vi "Dashboard Main.vi"() -> ()   [LabVIEW 2019]
uses:
  <vilib>/Rock Robotics/Network Tables/NT Read Numeric Array.vi
  <vilib>/Rock Robotics/Network Tables/NT Read String.vi
  <vilib>/Rock Robotics/Network Tables/NT Read Number.vi
  <vilib>/Rock Robotics/Network Tables/NT Read Boolean.vi
  <vilib>/Rock Robotics/Network Tables/NT Write Number.vi
panel:
  out "Camera Perf":string
  in  "Camera Settings":T1={"Frame Rate"=30, "Compression"=30, "Size"=1, "DB Camera Config"=FALSE} {"Frame Rate" scale=1.0..30.0; "Compression" scale=100.0..-1.0; "Size" items=["640x480", "320x240", "160x120"]}
  in  "TCP":refnum<k5>
  out "Robot IP":string
  in  "Dashboard Tab":T2(tab)
  in  "Select Auto":string(combo)="Select Autonomous ..."
  out "NT Connection":bool
  out "MotorChart R":cluster{"Numeric":dbl, "Numeric":dbl}(graph)
  out "MotorChart L":cluster{"Numeric":dbl, "Numeric":dbl}(graph)
  out "MotorSliders R":cluster{"MotorSlide1":dbl, "MotorSlide2":dbl} {"MotorSlide2" scale=-1.0..1.0 scale format="%#_2e"; "MotorSlide1" scale=-1.0..1.0 scale format="%#_2e"}
  out "MotorSliders L":cluster{"MotorSlide1":dbl, "MotorSlide2":dbl} {"MotorSlide2" scale=-1.0..1.0 scale format="%#_2e"; "MotorSlide1" scale=-1.0..1.0 scale format="%#_2e"}
  out "JS1 Z":dbl(slide) scale=-1.0..1.0 scale format="%#_2e"
  out "JS1 Graph":cluster{"X":dbl, "Y":dbl}[](graph)
  out "JS1 Buttons":T3
  out "JS2 Z":dbl(slide) scale=-1.0..1.0 scale format="%#_2e"
  out "JS2 Graph":cluster{"X":dbl, "Y":dbl}[](graph)
  out "JS2 Buttons":T3
  out "Mode":T4(ring)=enum."Auto Disabled"
  in  "Camera Name 2":string(combo)="No Camera Selection"
  out "Camera Image 2":T5(plugin-control)
  out "Target Spotted":bool
  out "Color Box":u32(colorbox)
  out "New Center Y":dbl
  out "New Center X":dbl
  out "y change":dbl
  out "Top Left Y":dbl
  out "Bottom Right Y":dbl
  out "Bottom Right X":dbl
  out "Top left X":dbl
  out "x change":dbl
  out "full angle":dbl
  in  "RectHeight":dbl
  in  "RectWidth":dbl
  in  "RectAngle":dbl
  in  "RectY":dbl
  in  "RectX":dbl
  out "Distance Formula 2":dbl
  out "Distance Formula 1":dbl
  out "Bottom Left Y":dbl
  out "Bottom Left X":dbl
  out "Top Right X":dbl
  out "Top Right Y":dbl
  out "New Full Angle":dbl
  out "2nd Y Change":dbl
  out "2nd X Change":dbl
  out "Final Center Y":dbl
  out "Final Center X":dbl
  out "Robot Angle":dbl
  out "Right Target":dbl
  out "Left Target":dbl
  out "Average Distance":dbl
  out "Right Distance":dbl
  out "Left Distance":dbl
  out "Right Speed":dbl
  out "Average Speed":dbl
  out "Left Speed":dbl
  out "Left":dbl[](graph)
  out "Right":dbl[](graph)
  out "Current Filter":T6 {"Value" scale=0.0..255.0; "Saturation" scale=0.0..255.0; "Hue" scale=0.0..255.0}
  in  "Update Filter":bool
  in  "New Filter":T6 {"Value" scale=0.0..255.0; "Saturation" scale=0.0..255.0; "Hue" scale=0.0..255.0}
  out "RectX":dbl
  out "RectY":dbl
  out "RectAngle":dbl
  out "RectWidth":dbl
  out "RectHeight":dbl
  out "left y":dbl
  out "right y":dbl
  out "right x":dbl
  out "left x":dbl
  out "right dmd":dbl format="%10.0f"
  out "lft dmd":dbl format="%10.0f"
  in  "Demand":bool
  in  "C Height":dbl format="%10.0f"
  in  "Update":bool
  in  "Kd":dbl format="%10.0f"
  in  "Ki":dbl format="%10.0f"
  in  "Kp":dbl format="%10.0f"
  in  "Kf":dbl format="%10.0f"
  out "Right Speed 2":dbl format="%10.0f"
  out "Left Speed 2":dbl format="%10.0f"
  out "Waveform Chart":dbl[](graph)
  in  "Right Dmd":dbl format="%10.0f"
  in  "Left Dmd":dbl format="%10.0f"
  out "Tree":string(tree)
  out "Camera Image":T5(plugin-control)
  out "Background":bool
  in  "Camera Name":string(combo)="No Camera Selection"
  # "HW"
  # "Joysticks"
  # "Drive Motors"
  # "Front"
  # "Right"
  # "Left"
  # "Back"
  # "Target Spotted"
  # "Color Sensor 90 Degree Color"
  # "Left"
  # "Right"
  # "Average"
  # "Speed"
  # "Target Speed"
  # "Distance"
  # "Robot Angle"
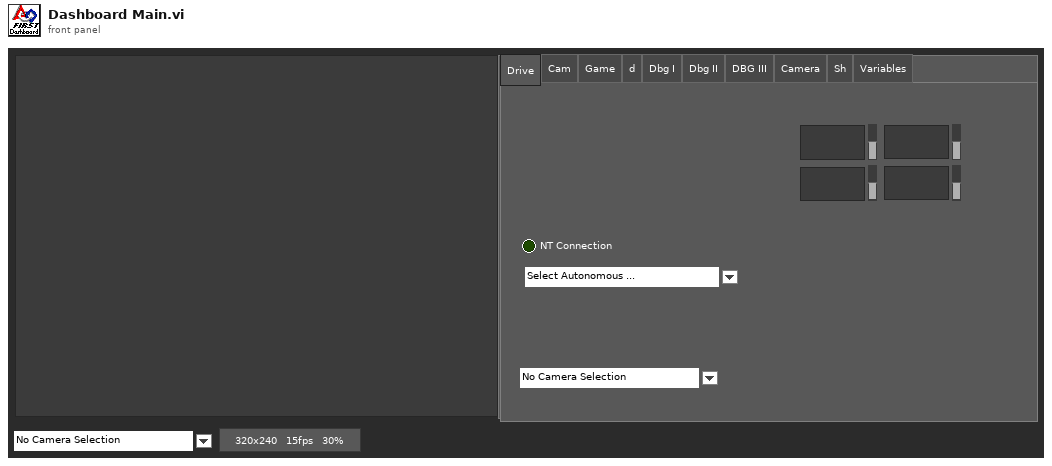
[diagram p1: front panel]
types:
  T1 = cluster{"Frame Rate":i32, "Compression":i32, "Size":u16, "DB Camera Config":bool}
  T2 = enum32{"Drive", "Cam", "Game", "d", "Dbg I", "Dbg II", "DBG III", "Camera", "Sh", "Variables"}
  T3 = cluster{bool, bool, bool, bool, bool, bool, bool, bool, bool, bool, bool, bool}
  T4 = enum8{"Tele-Op Disabled", "Tele-Op Enabled", "Auto Disabled", "Auto Enabled", "Test Disabled", "Test Enabled", "Disconnected", "No Code", "E-Stop"}
  T5 = typedef "IMAQ Image.ctl" = refnum<image>
  T6 = cluster{"Hue":cluster{dbl, dbl}, "Saturation":cluster{dbl, dbl}, "Value":cluster{dbl, dbl}}
  T7 = typedef "Image Type" = u32
  T8 = cluster{"Save Path":path, "Interval (s)":dbl, "Keep":i32}
  T9 = cluster{"Camera Image":refnum<vi>, "Dashboard Tab":refnum<vi>, "Background":refnum<vi>, "Tree":refnum<vi>, "Camera Settings":refnum<vi>, "Camera Name":refnum<vi>, "Camera Perf":refnum<vi>}
  T10 = cluster{"Shift":bool, "Ctrl":bool, "Alt":bool, "Cmd":bool, "Opt":bool}
  T11 = cluster{"Camera Name":string, "Camera File Name":string, "Saved DB Images Info":cluster{"Save Path":path, "Interval (s)":dbl, "Keep":i32}}
  T12 = cluster{"left x":dbl, "left y":dbl, "right x":dbl, "right y":dbl}
  T13 = cluster{cluster{dbl, dbl}, cluster{dbl, dbl}, cluster{dbl, dbl}}
  T14 = cluster{"left x":dbl, "right y":dbl, "right x":dbl, "left y":dbl}
  T15 = cluster{"Camera Name 2":string, string, "Saved DB Images Info":cluster{"Save Path":path, "Interval (s)":dbl, "Keep":i32}}
  T16 = cluster{"Error Strings":string, "Disable Counts":cluster{u16, u16}, "Rail Faults":cluster{u16, u16, u16}, "Robot IP":string, "DB Mode":u8, "Event Info":cluster{"Name":string, "Type":u8, "Number":u16, "Replay":u8}}
  T17 = cluster{"Storage":cluster{"Disk Free":u64, "RAM Block":u32, "RAM free":u32}, "CPU Utilization":cluster{"CPU % ISR":sgl, "CPU % Time Crit":sgl, "CPU % Timed Str":sgl, "CPU % High":sgl, "CPU % Above":sgl, "CPU % Normal":sgl, "CPU % Low":sgl}, "CAN":cluster{"% Bus Utilization":sgl, "Bus Off Cnt":u32, "TX_FIFO Full Cnt":u32, "Receive Error Cnt":u8, "Transmit Error Cnt":u8}, "HID":cluster{"HID Outputs":u32, "Rumble Low":u16, "Rumble High":u16}[]}
  T18 = cluster{"Status bits":cluster{"Test Mode":bool, "Autonomous":bool, "Enabled":bool, "Code Start":bool, "Brownout":bool, "Reserved 2":bool, "Reserved 3":bool, "E-Stop":bool}, "Code Trace":cluster{"Disabled":bool, "TeleOp":bool, "Auto":bool, "Test":bool}, "Controller Type":enum16{"unknown", "cRIO", "roboRio"}, "Code?":enum16{"unknown", "noCode", "code"}, "Battery V":dbl}
  T19 = cluster{"Control Bits":cluster{"TestMode":bool, "Autonomous":bool, "Enabled":bool, "FMS Present":bool, bool, bool, bool, "E-Stop":bool}, "Team Station ":u8, "Countdown":sgl, "Joystick Values":cluster{"Axes":dbl[], "Buttons":bool[], "POVs":i16[]}[]}
  T20 = cluster{"Axes":dbl[], "Buttons":bool[], "POVs":i16[]}[]
  T21 = cluster{"Axes":dbl[], "Buttons":bool[], "POVs":i16[]}
  T22 = cluster{"Buttons[0]":bool, "Buttons[1]":bool, "Buttons[2]":bool, "Buttons[3]":bool, "Buttons[4]":bool, "Buttons[5]":bool, "Buttons[6]":bool, "Buttons[7]":bool, "Buttons[8]":bool, "Buttons[9]":bool, "Buttons[10]":bool, "Buttons[11]":bool}
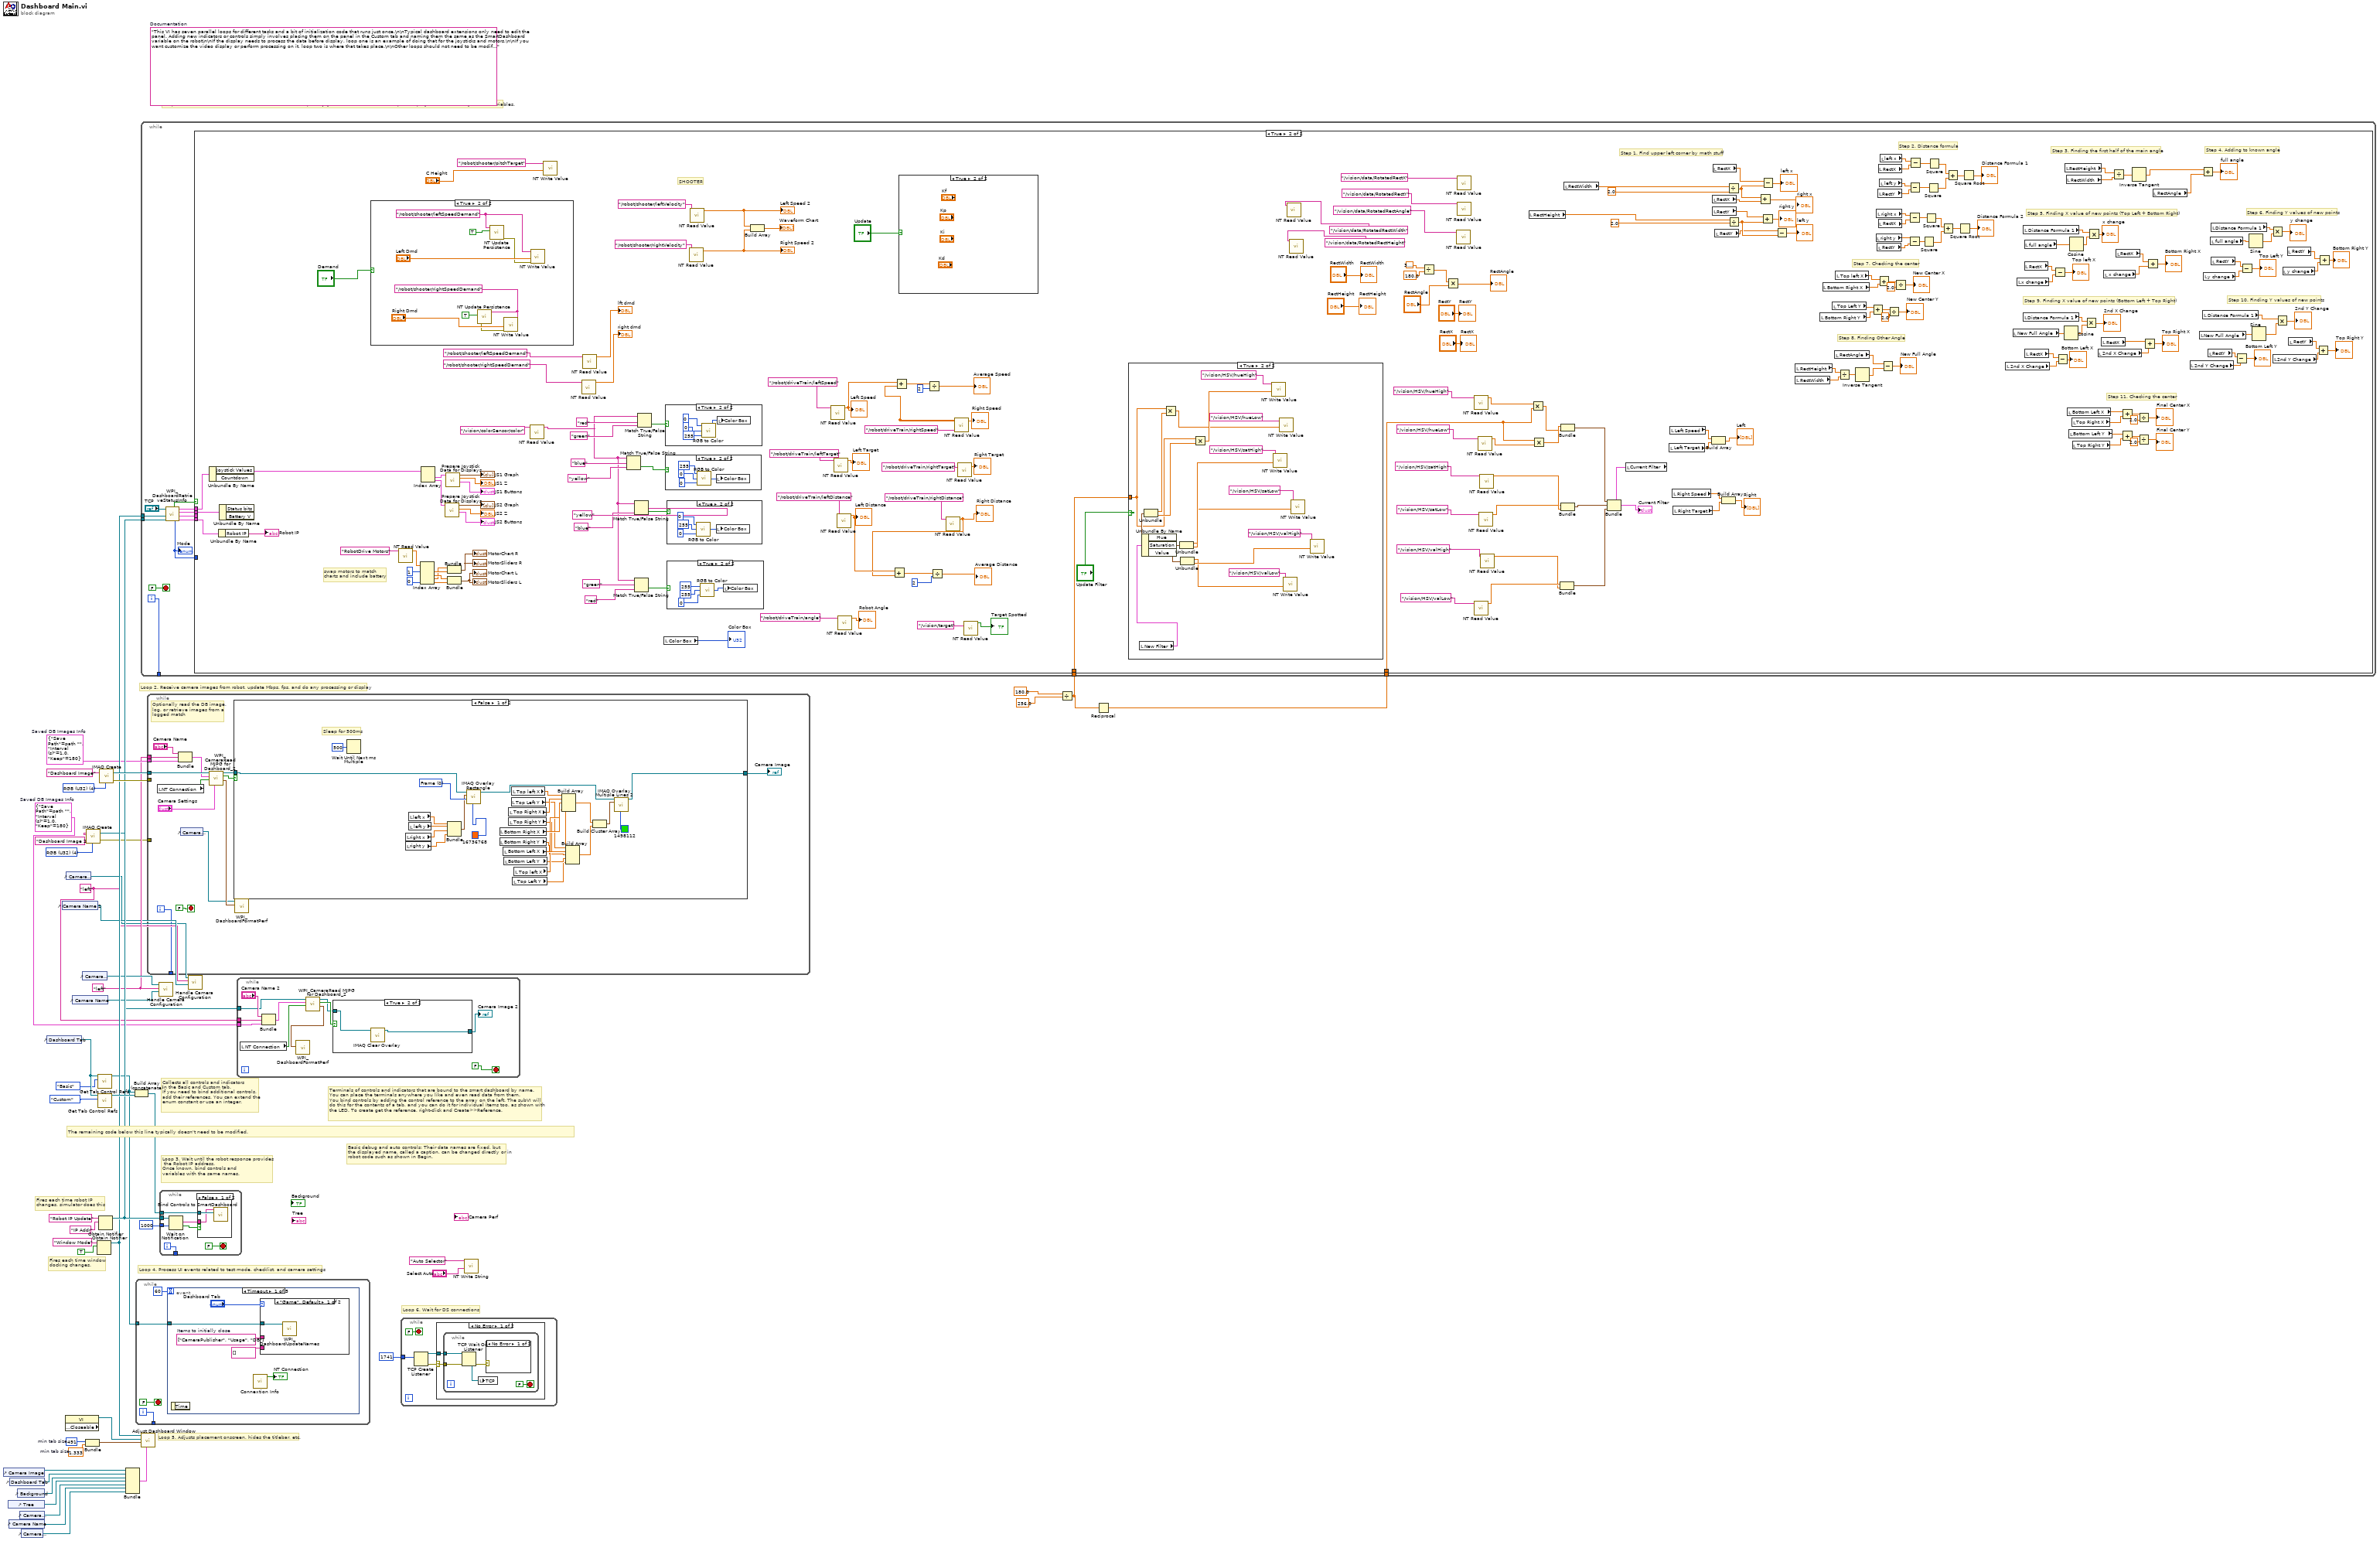
[diagram p0: block diagram]
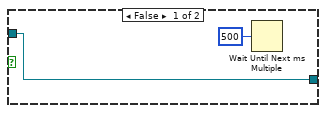
[diagram p2: hidden frame]
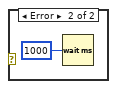
[diagram p3: hidden frame]
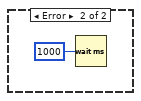
[diagram p4: hidden frame]
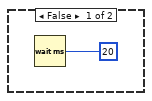
[diagram p5: hidden frame]
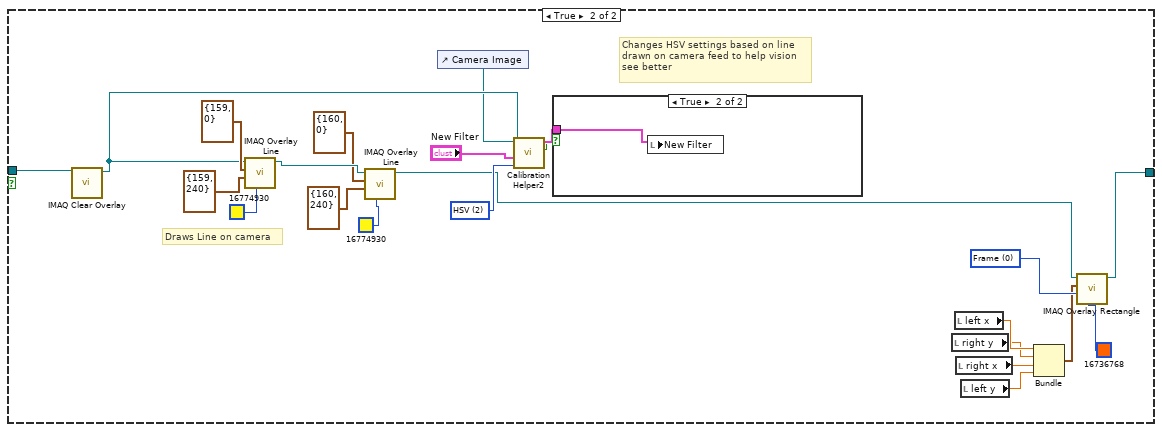
[diagram p14: hidden frame]
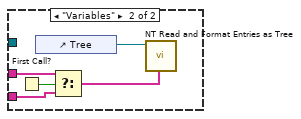
[diagram p16: hidden frame]
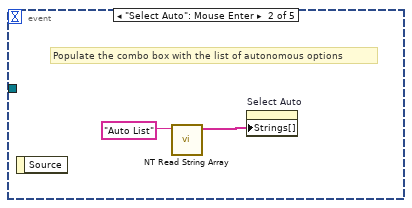
[diagram p17: hidden frame]
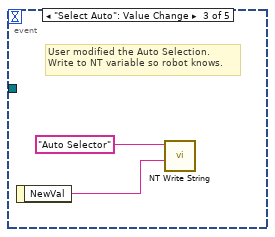
[diagram p18: hidden frame]
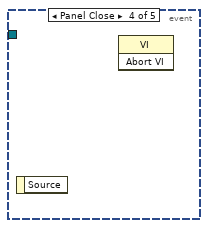
[diagram p19: hidden frame]
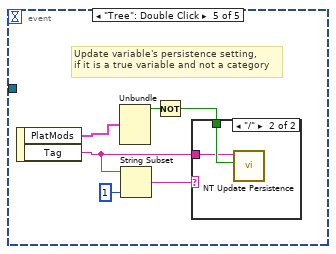
[diagram p20: hidden frame]
diagram:
  w5 = T7 4 items=["Grayscale (U8)", "Grayscale (I16)", "Grayscale (SGL)", "Complex (CSG)", "RGB (U32)", "HSL (U32)", "RGB (U64)"] ("Image Type")
  w2 = T8 {"Save Path"=path "", "Interval (s)"=1.0, "Keep"=180}  # Saved DB Images Info
  w3 = "left"
  w13 = "left" ("Camera File Name")
  w14 = T8 {"Save Path"=path "", "Interval (s)"=1.0, "Keep"=180}  # Saved DB Images Info
  w33 = 491  # min tab size
  w32 = 1.333  # min tab size
  (unwired) "This VI has seven parallel loops for different tasks and a bit of initialization code that runs just once.\n\nTypical dashboard extensions only need to edit the panel. Adding new indicators or controls simply involves placing them on the panel in the Custom tab and naming them the same as the SmartDashboard variable on the robot\n\nIf the display needs to process the data before display, loop one is an example of doing that for the joysticks and motors.\n\nIf you want customize the video display or perform processing on it, loop two is where that takes place.\n\nOther loops should not need to be modified. They are pretty standard, and document the task they perform."  # Documentation
  w48 = T7 4 items=["Grayscale (U8)", "Grayscale (I16)", "Grayscale (SGL)", "Complex (CSG)", "RGB (U32)", "HSL (U32)", "RGB (U64)"] ("Image Type")
  # "Terminals of controls and indicators that are bound to the smart dashboard by name.\nYou can place the terminals anywhere you like and even read data from them.\nYou bind controls by adding the control reference to the array on the left. The subVI will\ndo this for the contents of a tab, and you can do it for individual items too, as shown with\nthe LED. To create get the reference, right-click and Create>>Reference."
  # "Loop 6. Wait for DS connections"
  # "Basic debug and auto controls: Their data names are fixed, but\nthe displayed name, called a caption, can be changed directly or in\nrobot code such as shown in Begin."
  # "Fires each time robot IP\nchanges, simulator does this"
  # "Fires each time window\ndocking changes."
  # "Collects all controls and indicators\nin the Basic and Custom tab.\nIf you need to bind additional controls,\nadd their references. You can extend the\nenum constant or use an integer."
  # "The remaining code below this line typically doesn't need to be modified."
  # "Loop 4. Process UI events related to test mode, checklist, and camera settings"
  # "Loop 3. Wait until the robot response provides\n the Robot IP address.\nOnce known, bind controls and\nvariables with the same names."
  # "Loop 5. Adjusts placement onscreen, hides the titlebar, etc."
  # "Loop 1. Receive various data streams from Driver Station, update joystick, motors, and more complex displays that don't easily bind to variables."
  # "Loop 2. Receive camera images from robot, update Mbps, fps, and do any processing or display"
  n1 = control-ref of="Camera Image"() -> (w35:refnum<vi>)
  n2 = control-ref of="Tree"() -> (w20:refnum<vi>)
  n3 = control-ref of="Camera Name"() -> (w18:refnum<vi>)
  n4 = control-ref of="Dashboard Tab"() -> (w34:refnum<vi>)
  n5 = control-ref of="Background"() -> (w30:refnum<vi>)
  n6 = control-ref of="Camera Settings"() -> (w19:refnum<vi>)
  n7 = control-ref of="Camera Perf"() -> (w17:refnum<vi>)
  n8 = control-ref of="Dashboard Tab"() -> (w38:refnum<vi>)
  n9 = control-ref of="Camera Name 2"() -> (w8:refnum<vi>)
  n10 = property class="VI" props=["Front Panel.Closeable"]() -> (reference out=w39:refnum<vi>)  [unwired: 2 in, 2 out]
  n11 = control-ref of="Camera Settings"() -> (w7:refnum<vi>)
  n12 = control-ref of="Camera Name"() -> (w24:refnum<vi>)
  n13 = control-ref of="Camera Settings"() -> (w25:refnum<vi>)
  n14 = Bundle("min tab size"=w33, "min tab size"=w32) -> (w31:cluster{"min tab size":i32, "min tab size":dbl})  [unwired: 1 in]
  n15 = call "IMAQ Create"("Image Name"="Dashboard Image 2", "Image Type"=w5) -> ("New Image"=w1:T5, "error out"=w4:errorcluster)  [unwired: 2 in, 1 out]
  n16 = Obtain Notifier(name (unnamed)="Window Mode", notification data type=TRUE) -> (notifier out=w27:refnum<notifier>)  [unwired: 2 in, 2 out]
  n17 = call <vilib>:"Get Tab Control Refs.vi"("Page Index"=enum32{"Drive", "Basic", "Custom", "Variables"}."Basic" ("Dashboard Tab"), "TabControl in"=w38) -> ("ControlsOnPage"=w23:refnum<vi>[])  [unwired: 9 in]
  n18 = call <vilib>:"Get Tab Control Refs.vi"("Page Index"=enum32{"Drive", "Basic", "Custom", "Variables"}."Custom" ("Dashboard Tab"), "TabControl in"=w38) -> ("ControlsOnPage"=w37:refnum<vi>[])  [unwired: 9 in]
  n19 = Obtain Notifier(name (unnamed)="Robot IP Update", notification data type="IP Addr" ("name (unnamed)")) -> (notifier out=w28:refnum<notifier>)  [unwired: 2 in, 2 out]
  n20 = call "IMAQ Create"("Image Name"="Dashboard Image", "Image Type"=w48) -> ("New Image"=w46:T5, "error out"=w45:errorcluster)  [unwired: 2 in, 1 out]
  n21 = Bundle("Camera Image"=w35, "Dashboard Tab"=w34, "Background"=w30, "Tree"=w20, "Camera Settings"=w19, "Camera Name"=w18, "Camera Perf"=w17) -> (w29:T9)  [unwired: 1 in]
  n22 = Build Array (concatenate)(w23, w37) -> (w36:refnum<vi>[])
  n23 = while {
    tunnel: [w50] -> _
    tunnel: w23 -> [w49]
    i -> [w50]
    stop <- FALSE stop-if-true
    n24 = event shown="[0] Timeout" {
      selector: _ -> [_ _ _ _ _]
      dyn-events: _ -> [_ _ _ _ _]
      timeout: u32 60 ("milliseconds to wait") -> [_ _ _ _ _]
      tunnel: w49 -> [w55 _ _ _ _]
      event Timeout {
        w54 = string[] ["CameraPublisher", "Usage", "DB"]  # Items to initially close
        n25 = event-data() -> ()  [unwired: 1 in, 1 out]
        n26 = call <vilib>:"Connextion Info.vi"() -> ("Connected"=→"NT Connection":bool)  [unwired: 10 in, 1 out]
        n27 = case shown="\"Game\", Default" "Dashboard Tab" {
          tunnel: w55 -> [w58 _]
          tunnel: w54 -> [_ w61]
          tunnel: string[] [] -> [_ w60]
          frame "Game", Default {
            n28 = call <vilib>:"WPI_DashboardUpdateNames.vi"("Controls on Tab"=w58) -> ()  [unwired: 11 in]
          }
          frame "Variables" {
            n29 = First Call?() -> (First Call?: T/F=w62:bool)
            n30 = control-ref of="Tree"() -> (w63:refnum<vi>)
            n31 = Select(t=w61, s=w62, f=w60) -> (s? t:f=w59:string[])
            n32 = call <vilib>:"NT Read and Format Entries as Tree.vi"("Tags to  Close"=w59, "Tree Refnum"=w63) -> ()  [unwired: 8 in, 2 out]
          }
        }
      }
      event "Select Auto": Mouse Enter {
        # "Populate the combo box with the list of autonomous options"
        n33 = event-data() -> ()  [unwired: 1 in, 1 out]
        n34 = call <vilib>:"NT Read String Array.vi"("Name"="Auto List") -> ("String Array"=w64:string[])  [unwired: 9 in, 1 out]
        n35 = property on="Select Auto" class="CmbBox"("Strings[]"=w64) -> ()  [unwired: 2 in, 2 out]
      }
      event "Select Auto": Value Change {
        # "User modified the Auto Selection.\nWrite to NT variable so robot knows."
        n36 = event-data() -> ("NewVal"=w66:string)  [unwired: 1 in]
        n37 = call <vilib>:"NT Write String.vi"("String"=w66, "Name"="Auto Selector") -> ()  [unwired: 9 in, 1 out]
      }
      event Panel Close {
        n38 = event-data() -> ()  [unwired: 1 in, 1 out]
        n39 = invoke class="VI" method="Abort VI"() -> ()  [unwired: 3 in, 3 out]
      }
      event "Tree": Double Click {
        # "Update variable's persistence setting,\nif it is a true variable and not a category"
        n40 = event-data() -> ("PlatMods"=w69:T10, "Tag"=w68:string)  [unwired: 1 in]
        n41 = Unbundle(w69) -> ("Shift"=w73:bool)  [unwired: 4 out]
        n42 = String Subset(string=w68, length (rest)=1 ("length (rest)")) -> (substring=w70:string)  [unwired: 1 in]
        n43 = Not(x=w73) -> (.not. x?=w72:bool)
        n44 = case shown="\"/\"" w70 {
          tunnel: w72 -> [_ w75]
          tunnel: w68 -> [_ w74]
          frame Default {
          }
          frame "/" {
            n45 = call <vilib>:"NT Update Persistence.vi"("Persistence"=w75, "Name"=w74) -> ()  [unwired: 9 in, 1 out]
          }
        }
      }
    }
  }
  n46 = call "Adjust Dashboard Window.vi"("Sizing Refnums"=w29, "Size Constraints"=w31, "VI"=w39, "WIn Mode"=w27) -> ()  [unwired: 8 in]
  n47 = while {
    tunnel: w46 -> [w87]
    tunnel: w45 -> [_]
    tunnel: [w88] -> _
    tunnel: w14 -> [w82]
    tunnel: w13 -> [w79]
    tunnel: w4 -> [_]
    i -> [w88]
    stop <- FALSE stop-if-true
    # "Optionally read the DB image,\nlog, or retrieve images from a\nlogged match"
    n48 = local read "NT Connection"() -> (w83:bool)
    n49 = Bundle("Camera Name"="Camera Name", "Camera File Name"=w79, "Saved DB Images Info"=w82) -> (w81:T11)  [unwired: 1 in]
    n50 = control-ref of="Camera Perf"() -> (w77:refnum<vi>)
    n51 = call <vilib>:"WPI_CameraRead MJPG for Dashboard_2.vi"("Camera Settings"="Camera Settings", "NT Connection"=w83, "Capture Info"=w81, "Image in"=w87) -> ("perf info"=w78:cluster{"Bandwidth (Mbps)":dbl, "fps":dbl}, "Active"=w86:bool, "Image\\ out"=w76:T5)  [unwired: 5 in]
    n52 = case shown="False" w86 {
      tunnel: [w91 w117] -> w84
      tunnel: w76 -> [w112 w134]
      frame False {
        w113 = u32 0 items=["Frame", "Fill", "Highlight"] ("Drawing Mode (Frame)")
        # "Sleep for 500ms"
        n53 = Wait Until Next ms Multiple(millisecond multiple=u32 500) -> ()  [unwired: 1 out]
        n54 = local read "right x"() -> (w107:dbl)
        n55 = local read "right y"() -> (w106:dbl)
        n56 = local read "left x"() -> (w109:dbl)
        n57 = local read "left y"() -> (w108:dbl)
        n58 = Bundle("left x"=w109, "left y"=w108, "right x"=w107, "right y"=w106) -> (w110:T12)  [unwired: 1 in]
        n59 = call "IMAQ Overlay Rectangle"("Color"=u32 16736768, "Drawing Mode (Frame)"=w113, "Rectangle"=w110, "Image"=w112) -> ("Image Out"=w92:T5)  [unwired: 6 in, 1 out]
        n60 = local read "Bottom Right X"() -> (w103:dbl)
        n61 = local read "Bottom Right Y"() -> (w98:dbl)
        n62 = local read "Bottom Left X"() -> (w102:dbl)
        n63 = local read "Bottom Left Y"() -> (w97:dbl)
        n64 = local read "Top Right X"() -> (w104:dbl)
        n65 = local read "Top Right Y"() -> (w99:dbl)
        n66 = local read "Top Left Y"() -> (w100:dbl)
        n67 = local read "Top left X"() -> (w105:dbl)
        n68 = local read "Top Left Y"() -> (w96:dbl)
        n69 = local read "Top left X"() -> (w101:dbl)
        n70 = Build Array(w105, w104, w103, w102, w101) -> (w95:dbl[])
        n71 = Build Array(w100, w99, w98, w97, w96) -> (w94:dbl[])
        n72 = Build Cluster Array(w95, w94) -> (w93:cluster{"Top left X":dbl, "Top Left Y":dbl}[])
        n73 = call "IMAQ Overlay Multiple Lines 2"("Image"=w92, "Line End Points"=w93, "Color"=u32 1498112) -> ("Image Out"=w91:T5)  [unwired: 11 in, 1 out]
      }
      frame True {
        w124 = u32 0 items=["Frame", "Fill", "Highlight"] ("Drawing Mode (Frame)")
        w132 = u16 2 items=["RGB", "HSL", "HSV", "HSI", "CIE L*a*b*", "CIE XYZ"] ("Color Mode")
        # "Changes HSV settings based on line drawn on camera feed to help vision see better"
        # "Draws Line on camera"
        n74 = call "IMAQ Clear Overlay"("Image"=w134) -> ("Image Out"=w133:T5)  [unwired: 2 in, 8 out]
        n75 = call "IMAQ Overlay Line"("Color"=u32 16774930, "End Point"=cluster{i32, i32} {159, 240}, "Start Point"=cluster{i32, i32} {159, 0}, "Image"=w133) -> ("Image Out"=w128:T5)  [unwired: 6 in, 1 out]
        n76 = call "IMAQ Overlay Line"("Color"=u32 16774930, "End Point"=cluster{i32, i32} {160, 240}, "Start Point"=cluster{i32, i32} {160, 0}, "Image"=w128) -> ("Image Out"=w118:T5)  [unwired: 6 in, 1 out]
        n77 = control-ref of="Camera Image"() -> (w115:refnum<vi>)
        n78 = call "Calibration Helper2.vi"("Color Mode"=w132, "Color Components"="New Filter", "Image"=w133, "Image Ctl Refnum"=w115) -> ("Changed"=w130:bool, "output color"=w131:T13)  [unwired: 6 in]
        n79 = case shown="True" w130 {
          tunnel: w131 -> [_ w138]
          frame False {
          }
          frame True {
            n80 = local write "New Filter"(w138) -> ()
          }
        }
        n81 = local read "right y"() -> (w122:dbl)
        n82 = local read "left x"() -> (w123:dbl)
        n83 = local read "right x"() -> (w121:dbl)
        n84 = local read "left y"() -> (w120:dbl)
        n85 = Bundle("left x"=w123, "right y"=w122, "right x"=w121, "left y"=w120) -> (w119:T14)  [unwired: 1 in]
        n86 = call "IMAQ Overlay Rectangle"("Color"=u32 16736768, "Drawing Mode (Frame)"=w124, "Rectangle"=w119, "Image"=w118) -> ("Image Out"=w117:T5)  [unwired: 6 in, 1 out]
      }
    }
    "Camera Image" <- w84
    n87 = call <vilib>:"WPI_DashboardFormatPerf.vi"("Performance"=w78, "String in"=w77) -> ()  [unwired: 10 in]
  }
  n88 = call "Handle Camera Configuration.vi"("CameraNameRef"=w24, "Display Name"=w13, "ClusterRef"=w25) -> ()  [unwired: 9 in]
  n89 = while {
    tunnel: w36 -> [w145]
    tunnel: w28 -> [w143]
    tunnel: [w141] -> _
    tunnel: u32 1000 ("milliseconds to wait") -> [w140]
    i -> [w141]
    stop <- FALSE stop-if-true
    n90 = Wait on Notification(notifier=w143, timeout in ms (-1)=w140) -> (notification=w142:string, timed out?=w139:bool)  [unwired: 2 in, 2 out]
    n91 = case shown="False" w139 {
      tunnel: w145 -> [w147 _]
      tunnel: w142 -> [w146 _]
      frame False {
        n92 = call <vilib>:"Bind Controls to SmartDashboard.vi"("Bound Control Refs"=w147, "Server IP Address"=w146) -> ()  [unwired: 10 in]
      }
      frame True {
      }
    }
  }
  n93 = call "Handle Camera Configuration.vi"("CameraNameRef"=w8, "Display Name"=w3, "ClusterRef"=w7) -> ()  [unwired: 9 in]
  n94 = while {
    tunnel: w3 -> [w157]
    tunnel: w2 -> [w156]
    tunnel: w1 -> [w153]
    stop <- FALSE stop-if-true
    n95 = local read "NT Connection"() -> (w148:bool)
    n96 = Bundle("Camera Name 2"="Camera Name 2", w157, "Saved DB Images Info"=w156) -> (w154:T15)  [unwired: 1 in]
    n97 = call <vilib>:"WPI_CameraRead MJPG for Dashboard_2.vi"("NT Connection"=w148, "Capture Info"=w154, "Image in"=w153) -> ("perf info"=w149:cluster{"Bandwidth (Mbps)":dbl, "fps":dbl}, "Active"=w152:bool, "Image\\ out"=w151:T5)  [unwired: 6 in]
    n98 = call <vilib>:"WPI_DashboardFormatPerf.vi"("Performance"=w149) -> ()  [unwired: 11 in]
    n99 = case shown="True" w152 {
      tunnel: w151 -> [w159 w162]
      tunnel: [w159 w161] -> w150
      frame False {
        n100 = Wait Until Next ms Multiple(millisecond multiple=u32 500) -> ()  [unwired: 1 out]
      }
      frame True {
        n101 = call "IMAQ Clear Overlay"("Image"=w162) -> ("Image Out"=w161:T5)  [unwired: 2 in, 8 out]
      }
    }
    "Camera Image 2" <- w150
  }
  n102 = while {
    tunnel: u16 1741 ("timeout ms (25000)") -> [w164]
    stop <- FALSE stop-if-true
    n103 = TCP Create Listener(10:w164) -> (0:w163:errorcluster, 3:w165:refnum<k5>)  [unwired: 4 in, 1 out]
    n104 = case shown="No Error" w163 {
      selector: w163 -> [w167 _]
      tunnel: w165 -> [w168 _]
      frame No Error {
        n105 = while {
          tunnel: w168 -> [w171]
          tunnel: w167 -> [w170]
          stop <- FALSE stop-if-true
          n106 = TCP Wait On Listener(8:w170, 11:w171) -> (0:w172:errorcluster, 4:w173:refnum<k5>)  [unwired: 2 in, 3 out]
          n107 = local write "TCP"(w173) -> ()
          n108 = case shown="No Error" w172 {
            frame No Error {
            }
            frame Error {
              n109 = Wait (ms)(milliseconds to wait=u32 1000) -> ()  [unwired: 1 out]
            }
          }
        }
      }
      frame Error {
        n110 = Wait (ms)(milliseconds to wait=u32 1000) -> ()  [unwired: 1 out]
      }
    }
  }
  n111 = call <vilib>:"NT Write String.vi"("String"="Select Auto", "Name"="Auto Selector") -> ()  [unwired: 9 in, 1 out]
  n112 = Divide(x=180.0, y=256.0) -> (x/y=w10:dbl)
  n113 = Reciprocal(x=w10) -> (1/x=w9:dbl)
  n114 = while {
    tunnel: [w187] -> _
    tunnel: w28 -> [w181]
    tunnel: w27 -> [w178]
    tunnel: w10 -> [w177]
    tunnel: w9 -> [w176]
    i -> [w187]
    stop <- FALSE stop-if-true
    n115 = call <vilib>:"WPI_DashboardRetrieveStatusInfo.vi"("Binding Refnum"=w181, "Window Mode Notifier"=w178, "TCP Cnx"="TCP") -> ("Power and Errors"=w182:T16, "Robot Metrics"=w185:T17, "Status Info"=w186:T18, "Control Info"=w183:T19, "Robot Mode"=w180:T4, "Process?"=w184:bool)  [unwired: 3 in]
    "Mode" <- w180
    n116 = case shown="True" w184 {
      tunnel: w186 -> [_ w410]
      tunnel: w185 -> [_ _]
      tunnel: w183 -> [_ w409]
      tunnel: w182 -> [_ w408]
      tunnel: w180 -> [_ _]
      tunnel: w177 -> [_ w349]
      tunnel: w176 -> [_ w340]
      frame False {
        n117 = Wait (ms)(milliseconds to wait=u32 20) -> ()  [unwired: 1 out]
      }
      frame True {
        # "Step 11. Checking the center"
        # "Step 10. Finding Y values of new points"
        # "Step 9. Finding X value of new points (Bottom Left + Top Right)"
        # "Step 8. Finding Other Angle"
        # "Step 7. Checking the center"
        # "Step 6. Finding Y values of new points"
        # "Step 5. Finding X value of new points (Top Left + Bottom Right)"
        # "Step 4. Adding to known angle"
        # "Step 3. Finding the first half of the main angle"
        # "Step 2. Distance formula"
        # "Step 1. Find upper left corner by math stuff"
        # "SHOOTER"
        # "swap motors to match\ncharts and include battery"
        n118 = Unbundle By Name(w409) -> ("Joystick Values"=w399:T20)  [unwired: 1 out]
        n119 = Unbundle By Name(w408) -> ("Robot IP"=→"Robot IP":string)
        n120 = Unbundle By Name(w410) -> ()  [unwired: 2 out]
        n121 = case shown="True" "Demand" {
          frame False {
          }
          frame True {
            w413 = "/robot/shooter/rightSpeedDemand" ("Name")
            w416 = "/robot/shooter/leftSpeedDemand" ("Name")
            n122 = call <vilib>:"NT Update Persistence.vi"("Persistence"=TRUE, "Name"=w413) -> ("error out"=w412:errorcluster)  [unwired: 9 in]
            n123 = call <vilib>:"NT Update Persistence.vi"("Persistence"=TRUE, "Name"=w416) -> ("error out"=w415:errorcluster)  [unwired: 9 in]
            n124 = call-poly <vilib>:"NT Write Value.vi"("error in"=w412, "Numeric"="Right Dmd", "Name"=w413) -> ()  [unwired: 8 in, 1 out]
            n125 = call-poly <vilib>:"NT Write Value.vi"("error in"=w415, "Numeric"="Left Dmd", "Name"=w416) -> ()  [unwired: 8 in, 1 out]
          }
        }
        n126 = call-poly <vilib>:"NT Read Value.vi"("Name"="RobotDrive Motors") -> ("Numeric Array"=w389:dbl[])  [unwired: 9 in, 1 out]
        n127 = Index Array(array=w389, index #1=1, index #4=0) -> (element #1=w403:dbl, element #2=w404:dbl, element #3=w402:dbl, element #4=w407:dbl)  [unwired: 2 in]
        n128 = Index Array(array=w399) -> (element #1=w398:T21, element #2=w394:T21)  [unwired: 2 in]
        n129 = call "Prepare Joystick Data for Displays.vi"("Joystick Values"=w394) -> ("Buttons"=→"JS2 Buttons":T22, "Z Axis"=→"JS2 Z":dbl, "Cartesian Data"=→"JS2 Graph":cluster{"X axis":dbl, "X axis":dbl}[])  [unwired: 8 in]
        n130 = call "Prepare Joystick Data for Displays.vi"("Joystick Values"=w398) -> ("Buttons"=→"JS1 Buttons":T22, "Z Axis"=→"JS1 Z":dbl, "Cartesian Data"=→"JS1 Graph":cluster{"X axis":dbl, "X axis":dbl}[])  [unwired: 8 in]
        n131 = Bundle("Numeric"=w402, "Numeric"=w403) -> (→"MotorChart R" →"MotorSliders R":cluster{"Numeric":dbl, "Numeric":dbl})  [unwired: 1 in]
        n132 = Bundle("Numeric"=w404, "Numeric"=w407) -> (→"MotorChart L" →"MotorSliders L":cluster{"Numeric":dbl, "Numeric":dbl})  [unwired: 1 in]
        n133 = call-poly <vilib>:"NT Read Value.vi"("Name"="/vision/colorSensor/color") -> ("String"=w350:string)  [unwired: 9 in, 1 out]
        n134 = call-poly <vilib>:"NT Write Value.vi"("Numeric"="C Height", "Name"="/robot/shooter/pitchTarget") -> ()  [unwired: 9 in, 1 out]
        n135 = call-poly <vilib>:"NT Read Value.vi"("Name"="/robot/shooter/rightSpeedDemand") -> ("Numeric"=→"right dmd":dbl)  [unwired: 9 in, 1 out]
        n136 = call-poly <vilib>:"NT Read Value.vi"("Name"="/robot/shooter/leftSpeedDemand") -> ("Numeric"=→"lft dmd":dbl)  [unwired: 9 in, 1 out]
        n137 = Match True/False String(2:"yellow" ("false string"), 3:"blue" ("true string"), 4:w350) -> (0:w376:bool)  [unwired: 1 out]
        n138 = Match True/False String(2:"blue" ("false string"), 3:"yellow" ("true string"), 4:w350) -> (0:w375:bool)  [unwired: 1 out]
        n139 = Match True/False String(2:"red" ("false string"), 3:"green" ("true string"), 4:w350) -> (0:w385:bool)  [unwired: 1 out]
        n140 = Match True/False String(2:"green" ("false string"), 3:"red" ("true string"), 4:w350) -> (0:w386:bool)  [unwired: 1 out]
        n141 = local read "Color Box"() -> (→"Color Box":u32)
        n142 = case shown="True" w386 {
          frame False {
          }
          frame True {
            n143 = call <vilib>:"RGB to Color.vi"("B"=255, "G"=0, "R"=0) -> ("Color"=w450:u32)
            n144 = local write "Color Box"(w450) -> ()
          }
        }
        n145 = case shown="True" w376 {
          frame False {
          }
          frame True {
            n146 = call <vilib>:"RGB to Color.vi"("B"=0, "G"=0, "R"=255) -> ("Color"=w442:u32)
            n147 = local write "Color Box"(w442) -> ()
          }
        }
        n148 = case shown="True" w375 {
          frame False {
          }
          frame True {
            n149 = call <vilib>:"RGB to Color.vi"("B"=0, "G"=255, "R"=0) -> ("Color"=w438:u32)
            n150 = local write "Color Box"(w438) -> ()
          }
        }
        n151 = case shown="True" w385 {
          frame False {
          }
          frame True {
            n152 = call <vilib>:"RGB to Color.vi"("B"=0, "G"=255, "R"=255) -> ("Color"=w446:u32)
            n153 = local write "Color Box"(w446) -> ()
          }
        }
        n154 = call-poly <vilib>:"NT Read Value.vi"("Name"="/robot/shooter/rightVelocity") -> ("Numeric"=w320:dbl)  [unwired: 9 in, 1 out]
        "Right Speed 2" <- w320
        n155 = call-poly <vilib>:"NT Read Value.vi"("Name"="/robot/shooter/leftVelocity") -> ("Numeric"=w321:dbl)  [unwired: 9 in, 1 out]
        "Left Speed 2" <- w321
        n156 = Build Array(w321, w320) -> (→"Waveform Chart":dbl[])
        n157 = call-poly <vilib>:"NT Read Value.vi"("Name"="/robot/driveTrain/leftSpeed") -> ("Numeric"=w365:dbl)  [unwired: 9 in, 1 out]
        "Left Speed" <- w365
        n158 = call-poly <vilib>:"NT Read Value.vi"("Name"="/robot/driveTrain/leftTarget") -> ("Numeric"=→"Left Target":dbl)  [unwired: 9 in, 1 out]
        n159 = call-poly <vilib>:"NT Read Value.vi"("Name"="/robot/driveTrain/leftDistance") -> ("Numeric"=w360:dbl)  [unwired: 9 in, 1 out]
        "Left Distance" <- w360
        n160 = call-poly <vilib>:"NT Read Value.vi"("Name"="/robot/driveTrain/angle") -> ("Numeric"=→"Robot Angle":dbl)  [unwired: 9 in, 1 out]
        n161 = case shown="True" "Update" {
          frame False {
          }
          frame True {
          }
        }
        n162 = call-poly <vilib>:"NT Read Value.vi"("Name"="/robot/driveTrain/rightDistance") -> ("Numeric"=w359:dbl)  [unwired: 9 in, 1 out]
        "Right Distance" <- w359
        n163 = Add(x=w360, y=w359) -> (x+y=w358:dbl)
        n164 = Divide(x=w358, y=2) -> (x/y=→"Average Distance":dbl)
        n165 = call-poly <vilib>:"NT Read Value.vi"("Name"="/robot/driveTrain/rightSpeed") -> ("Numeric"=w364:dbl)  [unwired: 9 in, 1 out]
        "Right Speed" <- w364
        n166 = Add(x=w365, y=w364) -> (x+y=w363:dbl)
        n167 = Divide(x=w363, y=2) -> (x/y=→"Average Speed":dbl)
        n168 = call-poly <vilib>:"NT Read Value.vi"("Name"="/robot/driveTrain/rightTarget") -> ("Numeric"=→"Right Target":dbl)  [unwired: 9 in, 1 out]
        n169 = call-poly <vilib>:"NT Read Value.vi"("Name"="/vision/target") -> ("Boolean"=→"Target Spotted":bool)  [unwired: 9 in, 1 out]
        n170 = case shown="True" "Update Filter" {
          tunnel: w349 -> [_ w426]
          frame False {
          }
          frame True {
            n171 = local read "New Filter"() -> (w425:T6)
            n172 = Unbundle By Name(w425) -> ("Hue"=w437:cluster{dbl, dbl}, "Saturation"=w436:cluster{dbl, dbl}, "Value"=w435:cluster{dbl, dbl})
            n173 = Unbundle(w437) -> (w428:dbl, w427:dbl)
            n174 = Multiply(x=w426, y=w428) -> (x*y=w423:dbl)
            n175 = Unbundle(w436) -> (w421:dbl, w422:dbl)
            n176 = Unbundle(w435) -> (w419:dbl, w420:dbl)
            n177 = Multiply(x=w426, y=w427) -> (x*y=w424:dbl)
            n178 = call-poly <vilib>:"NT Write Value.vi"("Numeric"=w424, "Name"="/vision/HSV/hueHigh") -> ()  [unwired: 9 in, 1 out]
            n179 = call-poly <vilib>:"NT Write Value.vi"("Numeric"=w422, "Name"="/vision/HSV/satHigh") -> ()  [unwired: 9 in, 1 out]
            n180 = call-poly <vilib>:"NT Write Value.vi"("Numeric"=w423, "Name"="/vision/HSV/hueLow") -> ()  [unwired: 9 in, 1 out]
            n181 = call-poly <vilib>:"NT Write Value.vi"("Numeric"=w419, "Name"="/vision/HSV/valLow") -> ()  [unwired: 9 in, 1 out]
            n182 = call-poly <vilib>:"NT Write Value.vi"("Numeric"=w421, "Name"="/vision/HSV/satLow") -> ()  [unwired: 9 in, 1 out]
            n183 = call-poly <vilib>:"NT Write Value.vi"("Numeric"=w420, "Name"="/vision/HSV/valHigh") -> ()  [unwired: 9 in, 1 out]
          }
        }
        n184 = call-poly <vilib>:"NT Read Value.vi"("Name"="/vision/data/RotatedRectWidth") -> ()  [unwired: 9 in, 2 out]
        n185 = call-poly <vilib>:"NT Read Value.vi"("Name"="/vision/data/RotatedRectHeight") -> ()  [unwired: 9 in, 2 out]
        n186 = Divide(x=3.141592653589793, y=180.0) -> (x/y=w266:dbl)
        n187 = Multiply(x=w266, y="RectAngle") -> (x*y=→"RectAngle":dbl)
        n188 = call-poly <vilib>:"NT Read Value.vi"("Name"="/vision/data/RotatedRectAngle") -> ()  [unwired: 9 in, 2 out]
        n189 = call-poly <vilib>:"NT Read Value.vi"("Name"="/vision/data/RotatedRectX") -> ()  [unwired: 9 in, 2 out]
        n190 = call-poly <vilib>:"NT Read Value.vi"("Name"="/vision/data/RotatedRectY") -> ()  [unwired: 9 in, 2 out]
        n191 = call-poly <vilib>:"NT Read Value.vi"("Name"="/vision/HSV/hueHigh") -> ("Numeric"=w342:dbl)  [unwired: 9 in, 1 out]
        n192 = call-poly <vilib>:"NT Read Value.vi"("Name"="/vision/HSV/valLow") -> ("Numeric"=w330:dbl)  [unwired: 9 in, 1 out]
        n193 = call-poly <vilib>:"NT Read Value.vi"("Name"="/vision/HSV/hueLow") -> ("Numeric"=w341:dbl)  [unwired: 9 in, 1 out]
        n194 = call-poly <vilib>:"NT Read Value.vi"("Name"="/vision/HSV/satLow") -> ("Numeric"=w331:dbl)  [unwired: 9 in, 1 out]
        n195 = call-poly <vilib>:"NT Read Value.vi"("Name"="/vision/HSV/satHigh") -> ("Numeric"=w332:dbl)  [unwired: 9 in, 1 out]
        n196 = call-poly <vilib>:"NT Read Value.vi"("Name"="/vision/HSV/valHigh") -> ("Numeric"=w329:dbl)  [unwired: 9 in, 1 out]
        n197 = local read "RectHeight"() -> (w300:dbl)
        n198 = Multiply(x=w342, y=w340) -> (x*y=w333:dbl)
        n199 = Multiply(x=w340, y=w341) -> (x*y=w334:dbl)
        n200 = Bundle("Numeric"=w330, "Numeric"=w329) -> (w335:cluster{"Numeric":dbl, "Numeric":dbl})  [unwired: 1 in]
        n201 = Bundle(w334, w333) -> (w337:cluster{dbl, dbl})  [unwired: 1 in]
        n202 = Bundle("Numeric"=w331, "Numeric"=w332) -> (w336:cluster{"Numeric":dbl, "Numeric":dbl})  [unwired: 1 in]
        n203 = local read "RectWidth"() -> (w301:dbl)
        n204 = local read "Current Filter"() -> (w338:T6)
        n205 = Bundle(cluster=w338, "Hue"=w337, "Saturation"=w336, "Value"=w335) -> (→"Current Filter":T6)
        n206 = local read "Left Target"() -> (w316:dbl)
        n207 = local read "Left Speed"() -> (w317:dbl)
        n208 = local read "Right Speed"() -> (w313:dbl)
        n209 = local read "Right Target"() -> (w314:dbl)
        n210 = Build Array(w317, w316) -> (→"Left":dbl[])
        n211 = local read "RectX"() -> (w307:dbl)
        n212 = local read "RectY"() -> (w304:dbl)
        n213 = local read "RectX"() -> (w302:dbl)
        n214 = local read "RectY"() -> (w303:dbl)
        n215 = Build Array(w313, w314) -> (→"Right":dbl[])
        n216 = Divide(x=w301, y=2.0) -> (x/y=w306:dbl)
        n217 = Divide(x=w300, y=2.0) -> (x/y=w305:dbl)
        n218 = Add(x=w306, y=w307) -> (x+y=→"right x":dbl)
        n219 = Add(x=w304, y=w305) -> (x+y=→"right y":dbl)
        n220 = Subtract(x=w302, y=w306) -> (x-y=→"left x":dbl)
        n221 = Subtract(x=w303, y=w305) -> (x-y=→"left y":dbl)
        n222 = local read "RectHeight"() -> (w230:dbl)
        n223 = local read "RectWidth"() -> (w232:dbl)
        n224 = local read "Bottom Right Y"() -> (w237:dbl)
        n225 = local read "Bottom Right X"() -> (w241:dbl)
        n226 = local read "Top Left Y"() -> (w238:dbl)
        n227 = local read "RectAngle"() -> (w229:dbl)
        n228 = local read "Top left X"() -> (w242:dbl)
        n229 = Divide(x=w230, y=w232) -> (x/y=w231:dbl)
        n230 = Inverse Tangent(1:w231) -> (0:w228:dbl)
        n231 = Add(x=w238, y=w237) -> (x+y=w236:dbl)
        n232 = local read "right y"() -> (w285:dbl)
        n233 = local read "right x"() -> (w287:dbl)
        n234 = local read "RectY"() -> (w284:dbl)
        n235 = Add(x=w242, y=w241) -> (x+y=w240:dbl)
        n236 = local read "RectY"() -> (w288:dbl)
        n237 = local read "RectX"() -> (w296:dbl)
        n238 = local read "RectX"() -> (w286:dbl)
        n239 = local read "left y"() -> (w295:dbl)
        n240 = local read "left x"() -> (w297:dbl)
        n241 = Subtract(x=w229, y=w228) -> (x-y=→"New Full Angle":dbl)
        n242 = Divide(x=w236, y=2.0) -> (x/y=→"New Center Y":dbl)
        n243 = Divide(x=w240, y=2.0) -> (x/y=→"New Center X":dbl)
        n244 = Subtract(x=w287, y=w286) -> (x-y=w283:dbl)
        n245 = Subtract(x=w285, y=w284) -> (x-y=w282:dbl)
        n246 = Subtract(x=w295, y=w288) -> (x-y=w293:dbl)
        n247 = Subtract(x=w297, y=w296) -> (x-y=w294:dbl)
        n248 = Square(x=w282) -> (x^2=w280:dbl)
        n249 = Square(x=w283) -> (x^2=w281:dbl)
        n250 = Square(x=w293) -> (x^2=w291:dbl)
        n251 = Square(x=w294) -> (x^2=w292:dbl)
        n252 = Add(x=w281, y=w280) -> (x+y=w279:dbl)
        n253 = Add(x=w292, y=w291) -> (x+y=w290:dbl)
        n254 = Square Root(x=w279) -> (sqrt(x)=→"Distance Formula 2":dbl)
        n255 = Square Root(x=w290) -> (sqrt(x)=→"Distance Formula 1":dbl)
        n256 = local read "2nd X Change"() -> (w221:dbl)
        n257 = local read "New Full Angle"() -> (w226:dbl)
        n258 = local read "x change"() -> (w257:dbl)
        n259 = local read "Distance Formula 1"() -> (w224:dbl)
        n260 = local read "Distance Formula 1"() -> (w262:dbl)
        n261 = local read "full angle"() -> (w261:dbl)
        n262 = local read "RectX"() -> (w258:dbl)
        n263 = local read "RectX"() -> (w222:dbl)
        n264 = Subtract(x=w258, y=w257) -> (x-y=→"Top left X":dbl)
        n265 = Subtract(x=w222, y=w221) -> (x-y=→"Bottom Left X":dbl)
        n266 = Cosine(x=w226) -> (cos(x)=w225:dbl)
        n267 = local read "RectHeight"() -> (w273:dbl)
        n268 = local read "RectWidth"() -> (w272:dbl)
        n269 = local read "Bottom Left X"() -> (w202:dbl)
        n270 = local read "Bottom Left Y"() -> (w199:dbl)
        n271 = Cosine(x=w261) -> (cos(x)=w260:dbl)
        n272 = local read "Top Right X"() -> (w200:dbl)
        n273 = local read "Top Right Y"() -> (w198:dbl)
        n274 = Multiply(x=w224, y=w225) -> (x*y=→"2nd X Change":dbl)
        n275 = Multiply(x=w262, y=w260) -> (x*y=→"x change":dbl)
        n276 = local read "2nd X Change"() -> (w219:dbl)
        n277 = local read "RectX"() -> (w218:dbl)
        n278 = local read "x change"() -> (w254:dbl)
        n279 = Divide(x=w273, y=w272) -> (x/y=w271:dbl)
        n280 = local read "RectX"() -> (w255:dbl)
        n281 = Add(x=w202, y=w200) -> (x+y=w206:dbl)
        n282 = Add(x=w199, y=w198) -> (x+y=w204:dbl)
        n283 = Inverse Tangent(1:w271) -> (0:w265:dbl)
        n284 = Divide(x=w206, y=2.0) -> (x/y=→"Final Center X":dbl)
        n285 = Divide(x=w204, y=2.0) -> (x/y=→"Final Center Y":dbl)
        n286 = Add(x=w218, y=w219) -> (x+y=→"Top Right X":dbl)
        n287 = Add(x=w255, y=w254) -> (x+y=→"Bottom Right X":dbl)
        n288 = local read "RectAngle"() -> (w264:dbl)
        n289 = local read "2nd Y Change"() -> (w211:dbl)
        n290 = local read "New Full Angle"() -> (w216:dbl)
        n291 = Add(x=w265, y=w264) -> (x+y=→"full angle":dbl)
        n292 = local read "Distance Formula 1"() -> (w214:dbl)
        n293 = local read "y change"() -> (w247:dbl)
        n294 = local read "RectY"() -> (w212:dbl)
        n295 = local read "full angle"() -> (w250:dbl)
        n296 = local read "Distance Formula 1"() -> (w252:dbl)
        n297 = local read "RectY"() -> (w248:dbl)
        n298 = Subtract(x=w212, y=w211) -> (x-y=→"Bottom Left Y":dbl)
        n299 = Subtract(x=w248, y=w247) -> (x-y=→"Top Left Y":dbl)
        n300 = Sine(x=w250) -> (sin(x)=w251:dbl)
        n301 = Sine(x=w216) -> (sin(x)=w215:dbl)
        n302 = Multiply(x=w252, y=w251) -> (x*y=→"y change":dbl)
        n303 = local read "2nd Y Change"() -> (w208:dbl)
        n304 = Multiply(x=w214, y=w215) -> (x*y=→"2nd Y Change":dbl)
        n305 = local read "y change"() -> (w244:dbl)
        n306 = local read "RectY"() -> (w245:dbl)
        n307 = local read "RectY"() -> (w209:dbl)
        n308 = Add(x=w209, y=w208) -> (x+y=→"Top Right Y":dbl)
        n309 = Add(x=w245, y=w244) -> (x+y=→"Bottom Right Y":dbl)
        "RectX" <- "RectX"
        "RectY" <- "RectY"
        "RectWidth" <- "RectWidth"
        "RectHeight" <- "RectHeight"
      }
    }
  }
